vi "Rising Edge Detector.vi"(1 "In":bool) -> (0 "Out":bool)   [LabVIEW 2025]
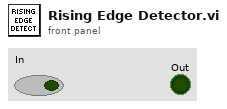
[diagram p1: front panel]
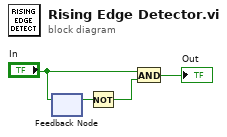
[diagram p0: block diagram]
diagram:
  n1 = feedback-in #1("In") -> ()
  n2 = feedback #1() -> (w3:bool)  [unwired: 1 in]
  n3 = Not(x=w3) -> (.not. x?=w4:bool)
  n4 = And(x="In", y=w4) -> (x .and. y?=→"Out":bool)
